vi "select MCS.vi"(8 "error in":errorcluster, 9 "idListSize":u32, 10 "idList":u32[](array[numeric]), 11 "UI SmarAct in":refnum<class "UI SmarAct.lvclass">) -> (0 "error out":errorcluster, 3 "UI SmarAct out":refnum<class "UI SmarAct.lvclass">)   [LabVIEW 2024, in "UI SmarAct.lvclass"]
doc: "Sélection du controleur MCS smaract"
uses:
  UI SmarAct.lvclass
  UI SmarAct.lvclass/UI SmarAct.ctl
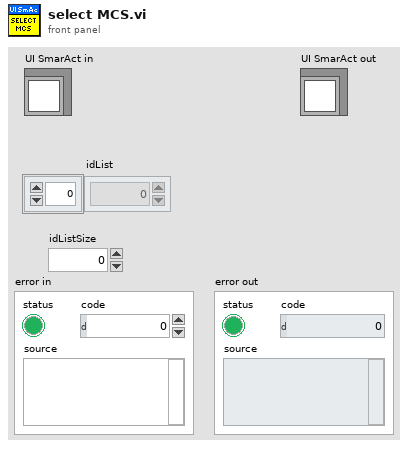
[diagram p1: front panel]
types:
  T1 = enum8{"Enabled", "Disabled", "Disabled and Grayed Out"}
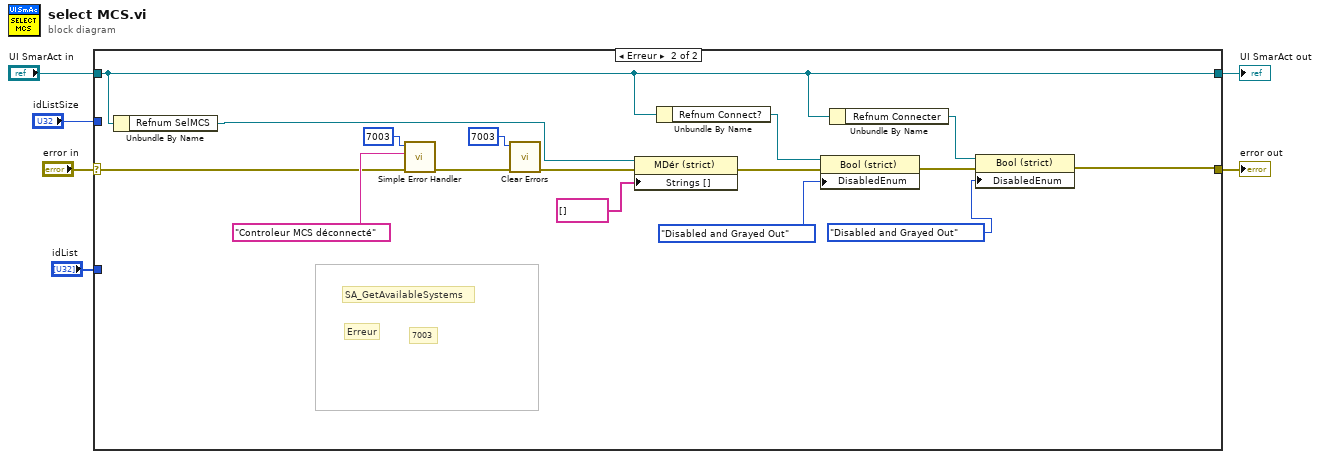
[diagram p0: block diagram]
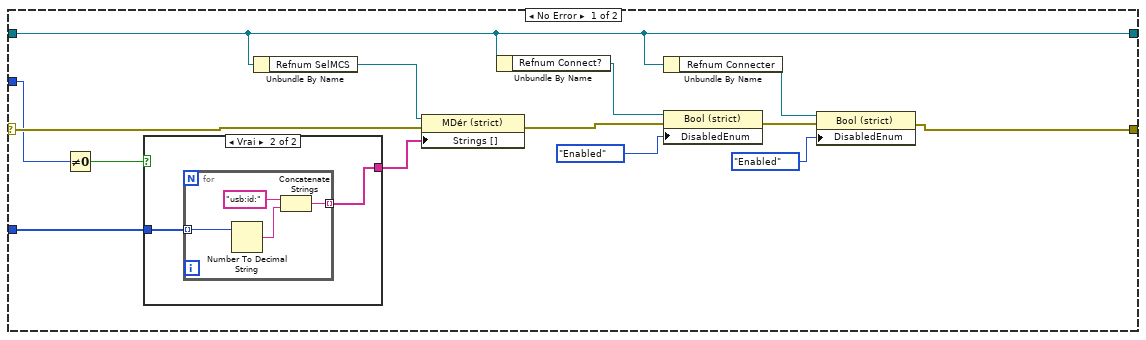
[diagram p2: hidden frame]
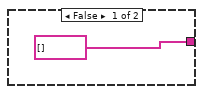
[diagram p3: hidden frame]
diagram:
  n1 = case shown="Erreur" "error in" {
    selector: "error in" -> [w18 w28]
    tunnel: [w11 w34] -> w6
    tunnel: "idList" -> [w19 _]
    tunnel: "idListSize" -> [w16 _]
    tunnel: "UI SmarAct in" -> [w9 w33]
    tunnel: [w9 w33] -> w2
    frame No Error {
      n2 = Not Equal To 0?(x=w16) -> (x != 0?=w20:bool)
      n3 = case shown="Vrai" w20 {
        tunnel: w19 -> [_ w22]
        tunnel: [string[] [] w23] -> w15
        frame False {
        }
        frame True {
          n4 = for {
            tunnel: [w25] -> w23 mode=indexing
            tunnel: w22 -> [w24] mode=indexing
            n5 = Number To Decimal String(number=w24) -> (decimal integer string=w27:string)  [unwired: 1 in]
            n6 = Concatenate Strings("usb:id:", w27) -> (w25:string)
          }
        }
      }
      n7 = Unbundle By Name(w9) -> ("Refnum SelMCS"=w17:refnum<vi>)
      n8 = property class="MDér (strict)"(reference=w17, error in=w18, "Strings []"=w15) -> (error out=w13:errorcluster)  [unwired: 1 out]
      n9 = Unbundle By Name(w9) -> ("Refnum Connect?"=w14:refnum<vi>)
      n10 = Unbundle By Name(w9) -> ("Refnum Connecter"=w10:refnum<vi>)
      n11 = property class="Bool (strict)"(reference=w14, error in=w13, "DisabledEnum"=T1."Enabled" ("Désactivée")) -> (error out=w12:errorcluster)  [unwired: 1 out]
      n12 = property class="Bool (strict)"(reference=w10, error in=w12, "DisabledEnum"=T1."Enabled" ("Désactivée")) -> (error out=w11:errorcluster)  [unwired: 1 out]
    }
    frame Error {
      # "Erreur"
      # "SA_GetAvailableSystems"
      # "7003"
      n13 = Unbundle By Name(w33) -> ("Refnum SelMCS"=w43:refnum<vi>)
      n14 = call <vilib>:"Simple Error Handler.vi"("error code (no error:0)"=7003, "error source (\" \")"="Controleur MCS déconnecté" ("error source (\" \")"), "error in (no error)"=w28) -> ("error out"=w42:errorcluster)  [unwired: 2 in, 4 out]
      n15 = call <vilib>:"Clear Errors.vi"("error in (no error)"=w42, "specific error code to clear (0: all)"=7003) -> ("error out"=w41:errorcluster)  [unwired: 4 in, 1 out]
      n16 = property class="MDér (strict)"(reference=w43, error in=w41, "Strings []"=string[] []) -> (error out=w35:errorcluster)  [unwired: 1 out]
      n17 = Unbundle By Name(w33) -> ("Refnum Connect?"=w31:refnum<vi>)
      n18 = property class="Bool (strict)"(reference=w31, error in=w35, "DisabledEnum"=T1."Disabled and Grayed Out" ("Désactivée")) -> (error out=w36:errorcluster)  [unwired: 1 out]
      n19 = Unbundle By Name(w33) -> ("Refnum Connecter"=w32:refnum<vi>)
      n20 = property class="Bool (strict)"(reference=w32, error in=w36, "DisabledEnum"=T1."Disabled and Grayed Out" ("Désactivée")) -> (error out=w34:errorcluster)  [unwired: 1 out]
    }
  }
  "error out" <- w6
  "UI SmarAct out" <- w2
